vi "DrawTable.vi"(8 "error in (no error)":errorcluster, 9 "Position":T1, 10 "GameIn":refnum<class "Game.lvclass">, 11 "Highscore in":refnum<class "Highscore.lvclass">) -> (0 "error out":errorcluster, 2 "GameOut":refnum<class "Game.lvclass">, 3 "Highscore out":refnum<class "Highscore.lvclass">)   [LabVIEW 2019, in "RT_Game.lvlib" / "Highscore.lvclass"]
uses:
  Highscore.lvclass
  Game/Coordinate.ctl
  Game/Game.lvclass
  Highscore.lvclass/Highscore.ctl
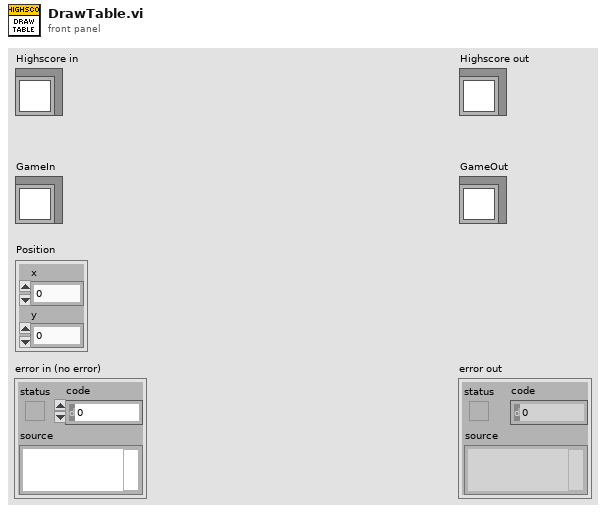
[diagram p1: front panel]
types:
  T1 = typedef "RT_Game.lvlib/Game.lvclass/Coordinate.ctl" = cluster{"x":dbl, "y":dbl}
  T2 = typedef "RT_Game.lvlib/Highscore.lvclass/HighscoreEntry.ctl" = cluster{"Name":string, "Score":dbl}
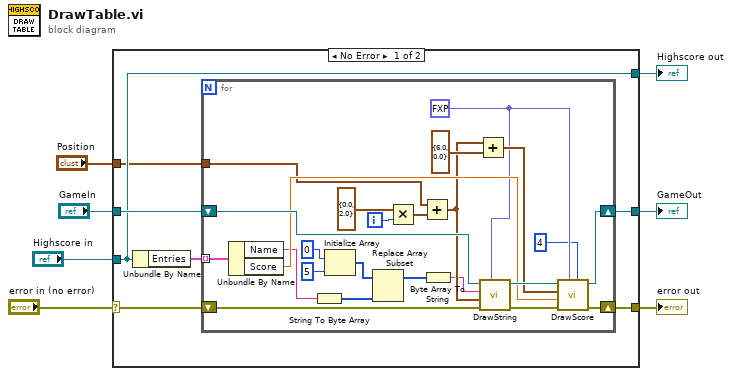
[diagram p0: block diagram]
diagram:
  n1 = case shown="No Error" "error in (no error)" {
    selector: "error in (no error)" -> [w14 w41]
    tunnel: [w13 w41] -> w6
    tunnel: [w10 w40] -> w4
    tunnel: "Highscore in" -> [w10 w40]
    tunnel: [w11 w39] -> w3
    tunnel: "GameIn" -> [w12 w39]
    tunnel: "Position" -> [w8 _]
    frame No Error {
      n2 = Unbundle By Name(w10) -> ("Entries"=w9:T2[])
      n3 = for {
        shift-right: [w35] -> w13
        shift-left: w14 -> [w38]
        shift-right: [w33] -> w11
        shift-left: w12 -> [w36]
        tunnel: w9 -> [w32] mode=indexing
        tunnel: w8 -> [w30]
        i -> [w22]
        w24 = fxp<+,3,3> 7.0 ("Color (7=white)")
        n4 = Unbundle By Name(w32) -> ("Name"=w18:string, "Score"=w31:dbl)
        n5 = String To Byte Array(string=w18) -> (unsigned byte array=w17:u8[])
        n6 = Initialize Array(u8 0 ("element"), 5 ("dimension size")) -> (w19:u8[])
        n7 = Replace Array Subset(array=w19, new element=w17) -> (w16:u8[])  [unwired: 1 in]
        n8 = Multiply(x=T1 {"x"=0.0, "y"=2.0}, y=w22) -> (x*y=w25:T1)
        n9 = Add(x=w30, y=w25) -> (x+y=w27:T1)
        n10 = Byte Array To String(unsigned byte array=w16) -> (string=w15:string)
        n11 = Add(x=w27, y=T1 {"x"=6.0, "y"=0.0}) -> (x+y=w28:T1)
        n12 = call "DrawString.vi"("Color (7=white)"=w24, "error in (no error)"=w38, "Coordinate"=w27, "String"=w15, "RT_Game.lvlib:Game.lvclass"=w36) -> ("error out"=w37:errorcluster, "RT_Game.lvlib:Game.lvclass 2"=w34:refnum<class "Game.lvclass">)  [unwired: 5 in]
        n13 = call "DrawScore.vi"("Digits"=4, "Color"=w24, "error in (no error)"=w37, "score"=w31, "position"=w28, "Pong in"=w34) -> ("error out"=w35:errorcluster, "Pong out"=w33:refnum<class "Game.lvclass">)  [unwired: 4 in]
      }
    }
    frame Error {
    }
  }
  "error out" <- w6
  "Highscore out" <- w4
  "GameOut" <- w3
